vi "ExSubCollectDisplayStoreQColor.vi"(0 "Handle Cluster":T2, 1 "Color Handle":u32, 2 "Display Title":string, 3 "Store flag":i8, 4 "Adjustments":T1={"Type of Bayer"=1, "Red Gain"=1.0, "Green Gain"=1.0, "Blue Gain"=1.0, "Bit shift"=0, "Red Offset"=0.0, "Green Offset"=0.0, "Blue Offset"=0.0} {"Blue Offset" format="%.2f"; "Green Offset" format="%.2f"; "Red Offset" format="%.2f"; "Blue Gain" format="%.2f"; "Green Gain" format="%.2f"; "Red Gain" format="%.2f"; "Type of Bayer" max=4 step=1}, 5 "error in (no error)":errorcluster) -> (6 "Handle Cluster Out":T2, 7 "got frame":u32, 8 "error out":errorcluster)   [LabVIEW 2012]
panel:
  # "ExSubCollectDisplayStoreCoolSnap:\nThis sub-VI checks to see if data has arrived from camera,\nif so it then puts it in image object and displays it. If store \nswitch is set it will also store it."
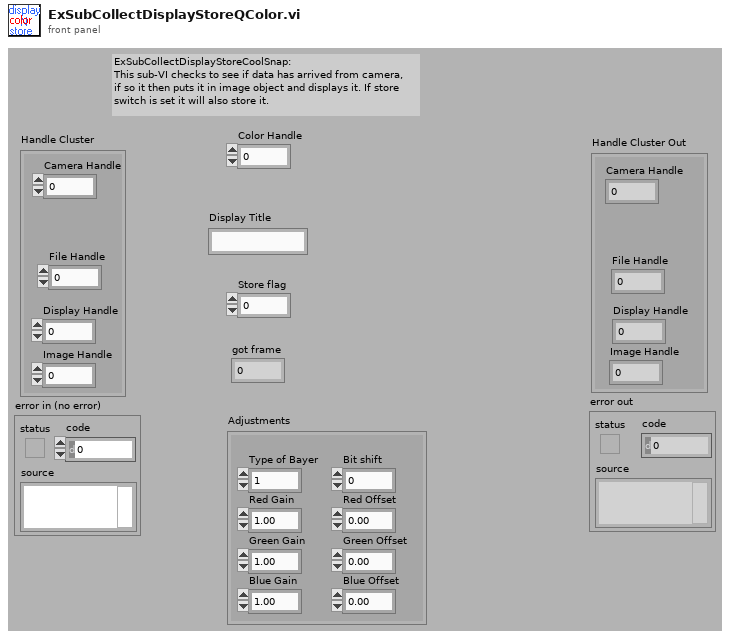
[diagram p1: front panel]
types:
  T1 = cluster{"Type of Bayer":u32, "Red Gain":dbl, "Green Gain":dbl, "Blue Gain":dbl, "Bit shift":u16, "Red Offset":dbl, "Green Offset":dbl, "Blue Offset":dbl}
  T2 = cluster{"Camera Handle":u32, "File Handle":u32, "Display Handle":u32, "Image Handle":u32}
  T3 = cluster{"Camera Handle":u32, "File Handle":u32, "Display Handle":u32, "RGB handle":u32}
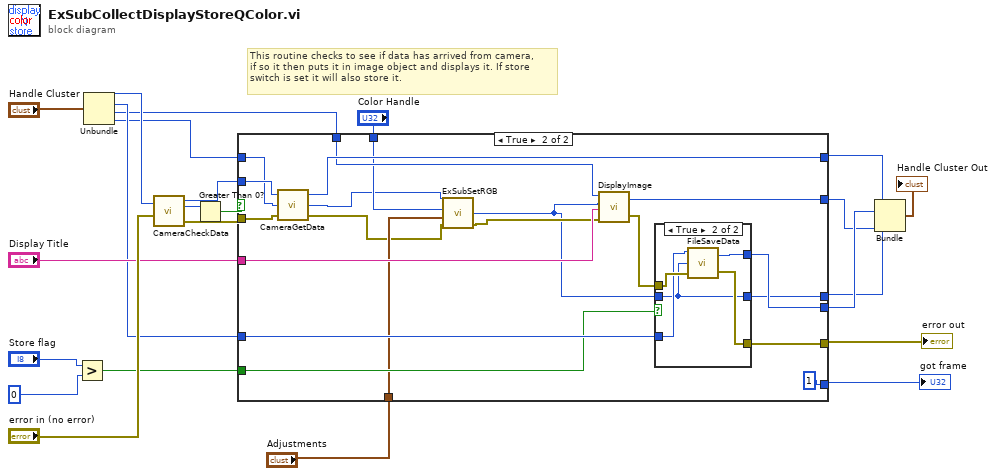
[diagram p0: block diagram]
diagram:
  # "This routine checks to see if data has arrived from camera,\nif so it then puts it in image object and displays it. If store \nswitch is set it will also store it."
  n1 = Greater?(x="Store flag", y=0) -> (0:w7:bool)
  n2 = Unbundle("Handle Cluster") -> ("Camera Handle"=w13:u32, "File Handle"=w5:u32, "Display Handle"=w4:u32, "Image Handle"=w3:u32)
  n3 = call <userlib>:"CameraCheckData.vi"("Camera Handle"=w13, "error in"="error in (no error)") -> ("Camera Handle"=w20:u32, "Number Of Frames Available"=w19:i32, "error out"=w18:errorcluster)
  n4 = Greater Than 0?(x=w19) -> (x > 0?=w21:bool)
  n5 = case shown="True" w21 {
    tunnel: w20 -> [w29 w49]
    tunnel: w18 -> [w28 w48]
    tunnel: w3 -> [w25 w44]
    tunnel: w4 -> [w27 w43]
    tunnel: [w29 w47] -> w14
    tunnel: [w26 w46] -> w12
    tunnel: "Display Title" -> [_ w42]
    tunnel: w5 -> [w26 w41]
    tunnel: [w27 w40] -> w11
    tunnel: [w28 w39] -> w15
    tunnel: [w25 w38] -> w10
    tunnel: w7 -> [_ w37]
    tunnel: [0 1] -> w6
    tunnel: "Adjustments" -> [_ w35]
    tunnel: "Color Handle" -> [_ w32]
    frame False {
    }
    frame True {
      n6 = call <userlib>:"CameraGetData.vi"("error in"=w48, "Image/Data Handle"=w44, "Camera Handle"=w49) -> ("error out"=w34:errorcluster, "Image/Data Handle"=w31:u32, "Camera Handle"=w47:u32)
      n7 = call "ExSubSetRGB.vi"("error in (no error)"=w34, "Adjustments"=w35, "RGB Handle"=w32, "Image handle"=w31) -> ("error out"=w33:errorcluster, "RGB handle"=w30:u32)  [unwired: 1 out]
      n8 = call <userlib>:"DisplayImage.vi"("error in"=w33, "Title"=w42, "Image Handle"=w30, "Display Handle"=w43) -> ("error out"=w45:errorcluster, "Display Handle"=w40:u32)
      n9 = case shown="True" w37 {
        tunnel: [w52 w57] -> w46
        tunnel: w45 -> [w51 w56]
        tunnel: w41 -> [w52 w54]
        tunnel: [w51 w55] -> w39
        tunnel: w30 -> [w50 w53]
        tunnel: [w50 w53] -> w38
        frame False {
        }
        frame True {
          n10 = call <userlib>:"FileSaveData.vi"("error in"=w56, "Image Handle"=w53, "File Handle"=w54) -> ("error out"=w55:errorcluster, "File Handle"=w57:u32)
        }
      }
    }
  }
  "error out" <- w15
  "got frame" <- w6
  n11 = Bundle("Camera Handle"=w14, "File Handle"=w12, "Display Handle"=w11, "RGB handle"=w10) -> (→"Handle Cluster Out":T3)  [unwired: 1 in]
